vi "File writing and analog testing.vi"() -> ()   [LabVIEW 2020]
doc: "This example demonstrates how to read N channels of analog input from a LINX device."
uses:
  <vilib>/MakerHub/LINX/Public/Peripherals/Analog/Analog Read N Chans.vi
  <vilib>/MakerHub/LINX/Private/Local IO/LinxAnalogRead.vi
  <vilib>/MakerHub/LINX/Public/Utilities/Check Channel.vi
  <vilib>/MakerHub/LINX/Public/Utilities/Open Serial.vi
  <vilib>/MakerHub/LINX/Private/Utilties/Generate Error.vi
  <vilib>/Analysis/Matrix/Numeric/Conversions/Array To Matrix - RA.vi
  <vilib>/Utility/file.llb/Write Delimited Spreadsheet (DBL).vi
  <vilib>/MakerHub/LINX/LMH-LINX.lvlib
  <vilib>/Analysis/Matrix/NI_Matrix.lvlib
panel:
  in  "?":T1(tab)
  in  "Serial Port":refnum<visa-resource-name>
  in  "Filename":string
  in  "File extension":string
  in  "Path":path
  out "Full filepath":string
  out "error out":errorcluster
  in  "?":bool
  out "WRITING TO FILE":bool
  in  "+      B":dbl
  in  "AX":dbl
  in  "Analog Port":dbl
  out "Time Stamp":timestamp
  out "Voltage":dbl
  out "Voltage":dbl(graph)
  out "Filtered Voltage":dbl(graph)
  out "Unfiltered Voltage":dbl
  out "Filtered Voltage":dbl
  out "Loop Rate (Hz)":u32
  in  "Stop Button":bool
  out "Pressure":dbl(graph)
  out "Pressure (PSI)":dbl
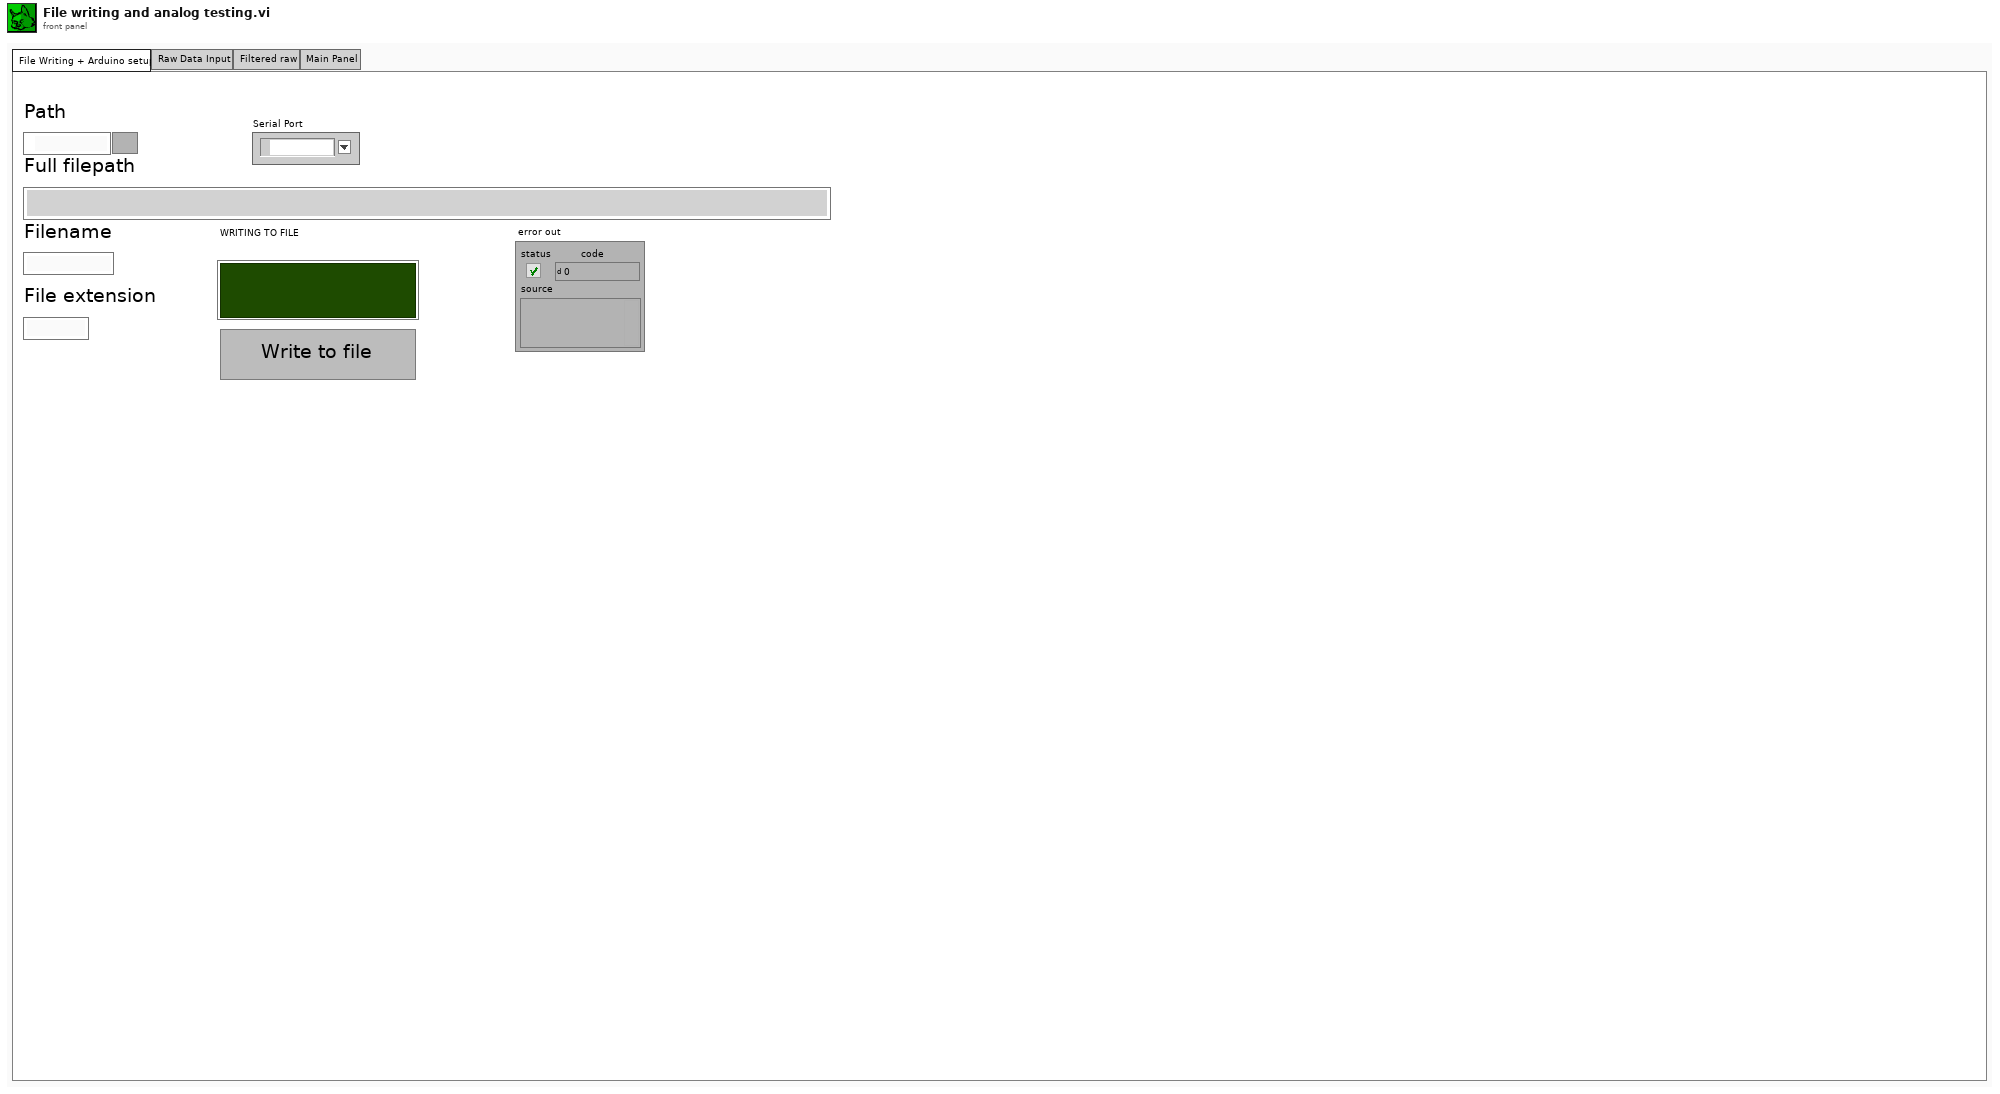
[diagram p1: front panel]
types:
  T1 = enum32{"File Writing + Arduino setup", "Raw Data Input", "Filtered raw", "Main Panel"}
  T2 = typedef "LMH-LINX.lvlib/LINX Ref.ctl" = cluster{"IO":T3, "Interface":T4, "LINX Device Config":T5}
  T3 = typedef "LMH-LINX.lvlib/Platform.ctl" = enum16{"Remote", "Local"}
  T4 = typedef "LMH-LINX.lvlib/Interface.ctl" = enum16{"Serial", "TCP"}
  T5 = typedef "LMH-LINX.lvlib/Device.lvlib/LINX Device Config.ctl" = cluster{"Interface":T4, "COM Port":refnum<visa-resource-name>, "TCP Configuration":T6, "Device Family":u8, "Device ID":u8, "Device Name":string, "TCP Ref":refnum<k5>, "Channels":T7}
  T6 = typedef "LMH-LINX.lvlib/Device.lvlib/TCP Config.ctl" = cluster{"IP Address":string, "Port":u16}
  T7 = typedef "LMH-LINX.lvlib/Channels.ctl" = cluster{"DI":u8[], "DO":u8[], "AI":u8[], "AO":u8[], "PWM":u8[], "QE":u8[], "UART":u8[], "I2C 2":u8[], "SPI":u8[], "CAN":u8[], "Servo":u8[], "AI Ref (V)":dbl, "AI Resolution (Bits)":u8, "AO Ref (V)":dbl, "AO Resolution (Bits)":u8}
  T8 = typedef "NI_Matrix.lvlib/RealMatrix.ctl" = dbl[][]
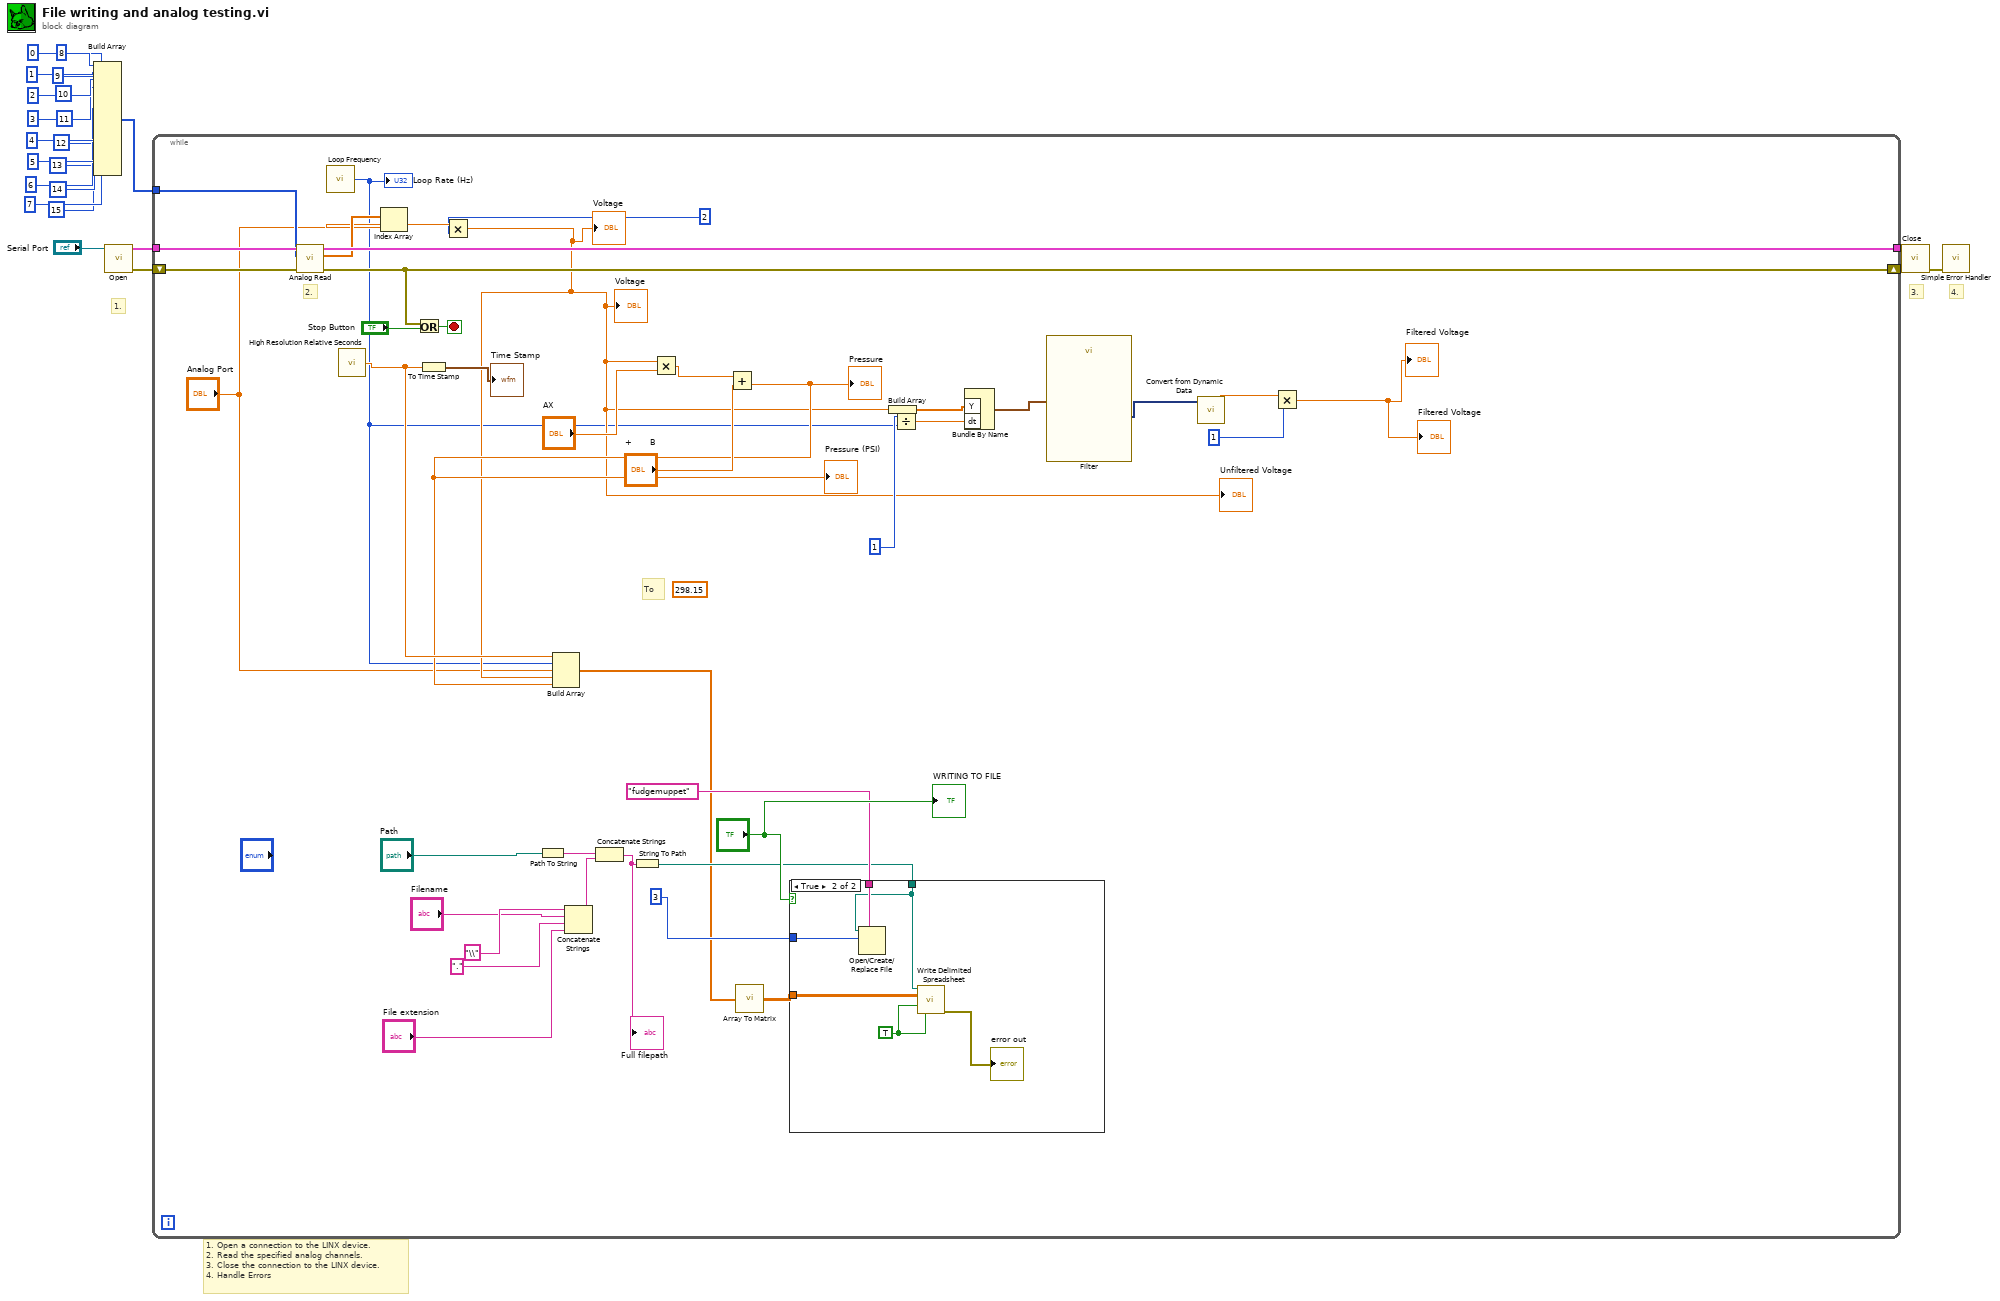
[diagram p0: block diagram]
diagram:
  # "1. Open a connection to the LINX device.\n2. Read the specified analog channels.\n3. Close the connection to the LINX device.\n4. Handle Errors"
  # "4."
  # "3."
  # "1."
  n1 = Build Array(0, 1, 2, 3, 4, 5, 6, 7, 8, 9, 10, 11, 12, 13, 14, 15) -> (w17:i32[])
  n2 = call-poly <vilib>:"Open.vi"("Serial Port"="Serial Port") -> ("Error Out"=w22:errorcluster, "LINX Resource"=w23:T2)  [unwired: 8 in, 1 out]
  n3 = while {
    tunnel: w23 -> [w64]
    tunnel: [w62] -> w21
    shift-right: [w59] -> w20
    shift-left: w22 -> [w63]
    tunnel: w17 -> [w58]
    stop <- w61 stop-if-true
    (unwired) 298.15
    # "To"
    # "2."
    n4 = call-poly <vilib>:"Analog Read.vi"("Error In"=w63, "AI Channel(s)"=w58, "LINX Resource"=w64) -> ("Error Out"=w59:errorcluster, "Voltages"=w57:dbl[], "LINX Resource"=w62:T2)  [unwired: 5 in, 1 out]
    n5 = call <vilib>:"Loop Frequency.vi"() -> ("Loop Rate (Hz)"=w38:u32)
    "Loop Rate (Hz)" <- w38
    n6 = call <vilib>:"High Resolution Relative Seconds.vi"() -> ("relative seconds"=w52:dbl)
    n7 = Index Array(array=w57, index="Analog Port") -> (element=w47:dbl)
    n8 = Or(x=w59, y="Stop Button") -> (x .or. y?=w61:bool)
    n9 = To Time Stamp(1:w52) -> (0:→"Time Stamp":timestamp)
    n10 = Multiply(x=w47, y=2) -> (x*y=w40:dbl)
    "Voltage" <- w40
    "Voltage" <- w40
    "Unfiltered Voltage" <- w40
    n11 = Path To String(path="Path") -> (string=w31:string)
    n12 = Concatenate Strings("\\", "Filename", ".", "File extension") -> (w24:string)
    n13 = Concatenate Strings(w31, w24) -> (w32:string)
    "Full filepath" <- w32
    n14 = String To Path(string=w32) -> (path=w33:path)
    n15 = Multiply(x=w40, y="AX") -> (x*y=w54:dbl)
    n16 = Add(x=w54, y="+      B") -> (x+y=w41:dbl)
    "Pressure" <- w41
    "Pressure (PSI)" <- w41
    n17 = Build Array(w52, w38, "Analog Port", w40, w41) -> (w29:dbl[])
    n18 = call-poly <vilib>:"Array To Matrix.vi"("Real 1D Array"=w29) -> ("Real Matrix (Column Vector)"=w37:T8)
    n19 = case shown="True" "?" {
      tunnel: w33 -> [_ w68]
      tunnel: w37 -> [_ w65]
      tunnel: "fudgemuppet" -> [_ w70]
      tunnel: 3 -> [_ w69]
      frame False {
      }
      frame True {
        w66 = TRUE
        n20 = Open/Create/Replace File(file path (use dialog)=w68, prompt=w70, operation (0:open)=w69) -> ()  [unwired: 3 in, 3 out]
        n21 = call-poly <vilib>:"Write Delimited Spreadsheet.vi"("file path (dialog if empty)"=w68, "2D data"=w65, "append to file? (new file:F)"=w66, "transpose? (no:F)"=w66) -> ("error out"=→"error out":errorcluster)  [unwired: 10 in, 1 out]
      }
    }
    n22 = Build Array(w40) -> (w49:dbl[])
    n23 = Divide(x=1, y=w38) -> (x/y=w51:dbl)
    n24 = Bundle By Name("Y"=w49, "dt"=w51) -> (w48:waveform(dbl))  [unwired: 1 in]
    n25 = call "Filter"("Signal"=w48) -> ("Filtered Signal"=w45:dynamicdata)  [unwired: 9 in, 1 out]
    n26 = call "Convert from Dynamic Data"("Dynamic Data Type"=w45) -> ("Scalar"=w44:dbl)  [unwired: 3 in]
    n27 = Multiply(x=w44, y=1) -> (x*y=→"Filtered Voltage" →"Filtered Voltage":dbl)
    "WRITING TO FILE" <- "?"
  }
  n28 = call <vilib>:"Close.vi"("Error In"=w20, "LINX Resource"=w21) -> ("Error Out"=w18:errorcluster)  [unwired: 9 in]
  n29 = call <vilib>:"Simple Error Handler.vi"("error in (no error)"=w18) -> ()  [unwired: 4 in, 5 out]
